vi "Processed Output Path.vi"(5 "Entrypoint (main)":string="main", 7 "Platform":string, 11 "Source Via Path":path) -> (2 "Processed Output Folder":path, 3 "Processed Output Path":path)   [LabVIEW 2020, in "PicoG-Processor.lvlib" / "GVIWebProcessorApp.lvclass"]
uses:
  GVIWebProcessorApp.lvclass
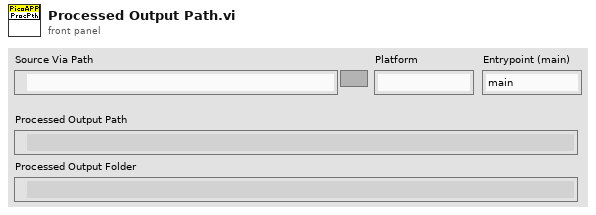
[diagram p1: front panel]
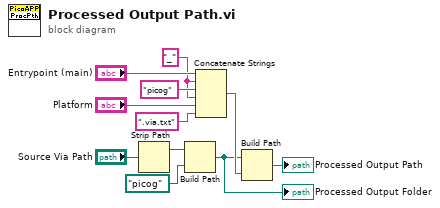
[diagram p0: block diagram]
diagram:
  w8 = "_" ("string")
  n1 = Strip Path(path="Source Via Path") -> (stripped path=w5:path)  [unwired: 1 out]
  n2 = Build Path(base path=w5, name or relative path=path "picog") -> (appended path=w1:path)
  "Processed Output Folder" <- w1
  n3 = Concatenate Strings("Entrypoint (main)", w8, "picog" ("string"), w8, "Platform", ".via.txt" ("string")) -> (w3:string)
  n4 = Build Path(base path=w1, name or relative path=w3) -> (appended path=→"Processed Output Path":path)
